vi "Close.vi"(8 "error in (no error)":errorcluster, 11 "Camera Imaqdx in":refnum<class "Camera Imaqdx.lvclass">) -> (0 "error out":errorcluster, 3 "Camera Imaqdx out":refnum<class "Camera Imaqdx.lvclass">)   [LabVIEW 2023]
uses:
  <vilib>/userDefined/High Color/IMAQdx.ctl
  Camera Imaqdx.lvclass
  D:/git/HAL/Camera Base/Camera Base.lvclass
  D:/git/HAL/Hardware_class/Instrument.lvclass
  D:/git/HAL/Interfaces/ICamera/ICamera.lvclass
  D:/git/HAL/Camera Imaqdx/Camera Imaqdx.lvclass
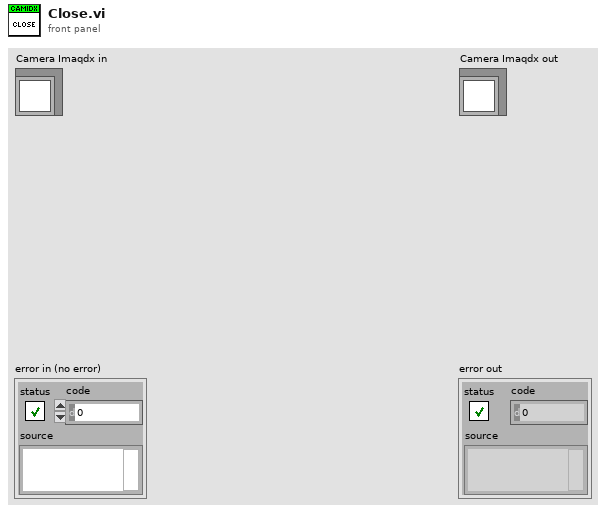
[diagram p1: front panel]
types:
  T1 = typedef "IMAQdx.ctl" = refnum<k21>
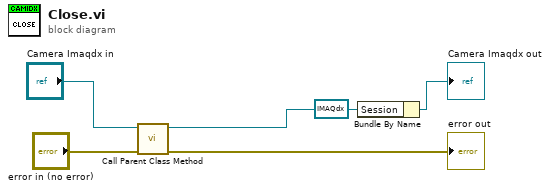
[diagram p0: block diagram]
diagram:
  n1 = call-parent "Call Parent Class Method"("error in (no error)"="error in (no error)", "Camera Base in"="Camera Imaqdx in") -> ("error out"=→"error out":errorcluster, "Camera Base out"=w3:refnum<class "Camera Imaqdx.lvclass">)  [unwired: 8 in]
  n2 = Bundle By Name(cluster=w3, "Session"=T1 refnum) -> (→"Camera Imaqdx out":refnum<class "Camera Imaqdx.lvclass">)
